vi "ENPH 354 Assignment 2 - Q4.vi"() -> ()   [LabVIEW 2021]
panel:
  out "XY Graph":cluster{dbl[], dbl[]}(graph)
  in  "Ball Speed Control":dbl(knob) scale=0.0..100.0
  in  "stop":bool
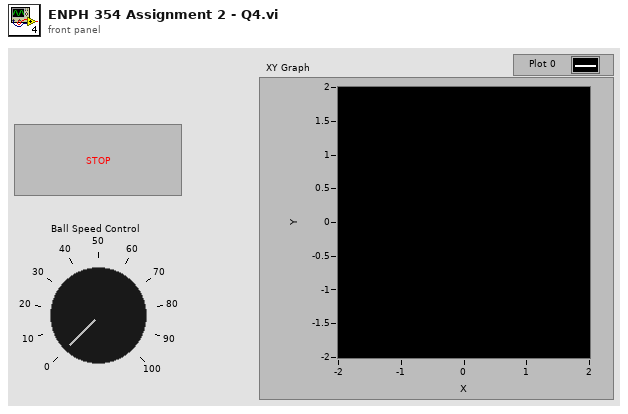
[diagram p1: front panel]
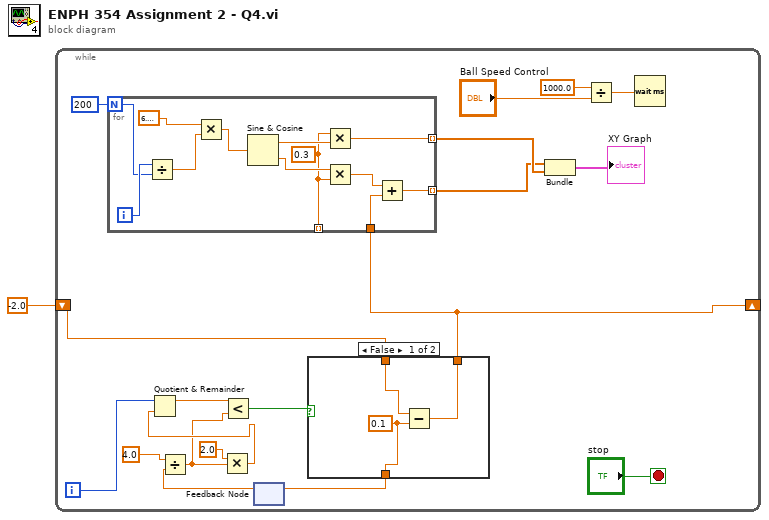
[diagram p0: block diagram]
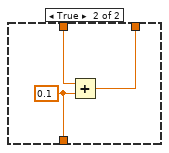
[diagram p2: hidden frame]
diagram:
  n1 = while {
    shift-right: [w11] -> _
    shift-left: -2.0 ("x") -> [w12]
    i -> [w10]
    stop <- "stop" stop-if-true
    n2 = feedback #1() -> (w2:dbl)  [unwired: 1 in]
    n3 = Divide(x=4.0, y=w2) -> (x/y=w4:dbl)
    n4 = Multiply(x=2.0, y=w4) -> (x*y=w5:dbl)
    n5 = Quotient & Remainder(x=w10, y=w5) -> (x-y*floor(x/y)=w8:dbl)  [unwired: 1 out]
    n6 = Less?(x=w8, y=w4) -> (x < y?=w6:bool)
    n7 = case shown="False" w6 {
      tunnel: w12 -> [w23 w26]
      tunnel: [w22 w25] -> w11
      tunnel: [w21 w24] -> w3
      frame False {
        w21 = 0.1 ("y")
        n8 = Subtract(x=w23, y=w21) -> (x-y=w22:dbl)
      }
      frame True {
        w24 = 0.1 ("y")
        n9 = Add(x=w26, y=w24) -> (x+y=w25:dbl)
      }
    }
    n10 = for {
      N: 200 -> [w37]
      tunnel: [w30] -> w13 mode=indexing
      tunnel: [w29] -> _ mode=indexing
      tunnel: [w28] -> w14 mode=indexing
      tunnel: w11 -> [w27]
      i -> [w38]
      w29 = 0.3 ("y")
      n11 = Divide(x=w38, y=w37) -> (x/y=w35:dbl)
      n12 = Multiply(x=6.283185307179586, y=w35) -> (x*y=w34:dbl)
      n13 = Sine & Cosine(0:w34) -> (1:w33:dbl, 2:w32:dbl)
      n14 = Multiply(x=w29, y=w33) -> (x*y=w28:dbl)
      n15 = Multiply(x=w32, y=w29) -> (x*y=w31:dbl)
      n16 = Add(x=w31, y=w27) -> (x+y=w30:dbl)
    }
    n17 = feedback-in #1(w3) -> ()
    n18 = Bundle(w13, w14) -> (→"XY Graph":cluster{dbl[], dbl[]})  [unwired: 1 in]
    n19 = Divide(x=1000.0, y="Ball Speed Control") -> (x/y=w16:dbl)
    n20 = Wait (ms)(milliseconds to wait=w16) -> ()  [unwired: 1 out]
  }
